vi "Save Image.vi"(8 "error in (no error)":errorcluster, 10 "Path":path, 11 "Camera Process in":refnum<class "Camera Process.lvclass">) -> (0 "error out":errorcluster, 3 "Camera Process out":refnum<class "Camera Process.lvclass">)   [LabVIEW 2022 SP3, in "Cam Process.lvlib" / "Camera Process.lvclass"]
uses:
  Camera Process.lvclass
  Camera Process.lvclass/Camera Process.ctl
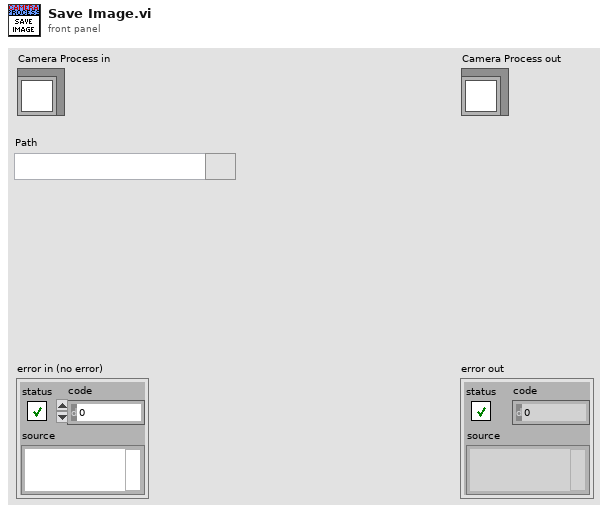
[diagram p1: front panel]
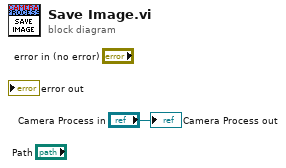
[diagram p0: block diagram]
diagram:
  "Camera Process out" <- "Camera Process in"
